vi "Get Service Class Instances.vi"() -> (3 "service instances":refnum<class "ServiceBase.lvclass">[](array[class]))   [LabVIEW 2025, in "Automotive-Vision-OOBService_server.lvlib"]
uses:
  Automotive-Vision-OOBService_server.lvlib
  <vilib>/gRPC/LabVIEW gRPC Servicer/ServiceBase/ServiceBase.lvclass
  RPC Service/ExamplePluginOOBService/ExamplePluginOOBService.lvclass
  C:/Program Files/National Instruments/LabVIEW 2025/vi.lib/gRPC/LabVIEW gRPC Servicer/ServiceBase/ServiceBase.lvclass
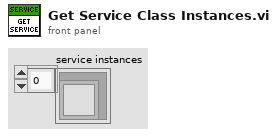
[diagram p1: front panel]
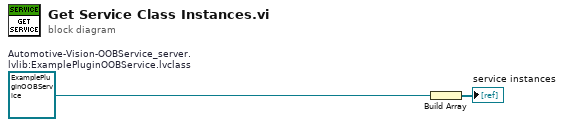
[diagram p0: block diagram]
diagram:
  w1 = refnum<class "ExamplePluginOOBService.lvclass"> refnum  # Automotive-Vision-OOBService_server.lvlib:ExamplePluginOOBService.lvclass
  n1 = Build Array(w1) -> (→"service instances":refnum<class "ExamplePluginOOBService.lvclass">[])
